vi "Straighten Array.vi"(8 "Error In":errorcluster, 11 "Array":dbl[](array[numeric])) -> (0 "Error Out":errorcluster, 3 "Straightened Array":dbl[](array[numeric]))   [LabVIEW 2021, in "Arrays.lvlib"]
doc: "Tries to make consecutive values monotonically increasing.\nWill fail if the last value is not the larges one."
uses:
  Arrays.lvlib
panel:
  out "Waveform Chart":T1(graph)
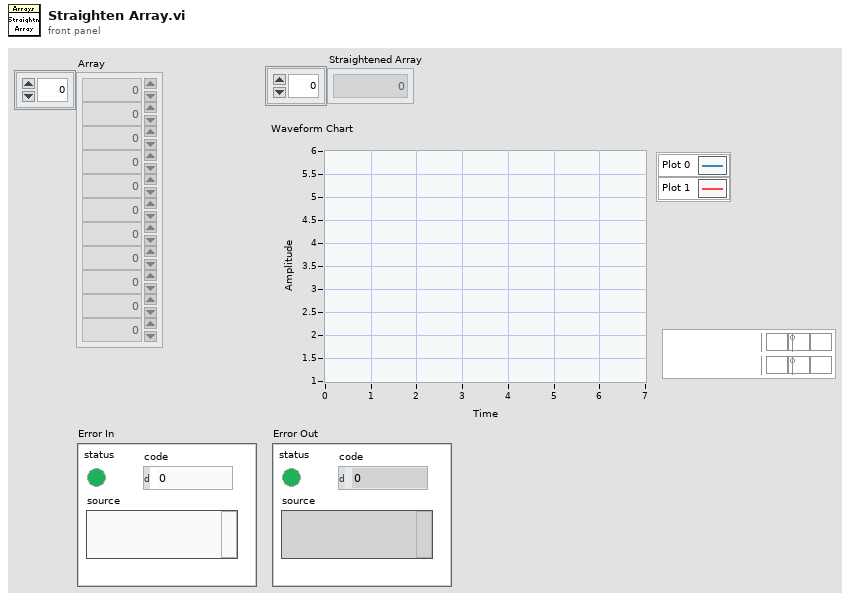
[diagram p1: front panel]
types:
  T1 = cluster{"Numeric Control":dbl, "Numeric Control":dbl}
  T2 = cluster{"Numeric Control":dbl, "Numeric Control":dbl}[]
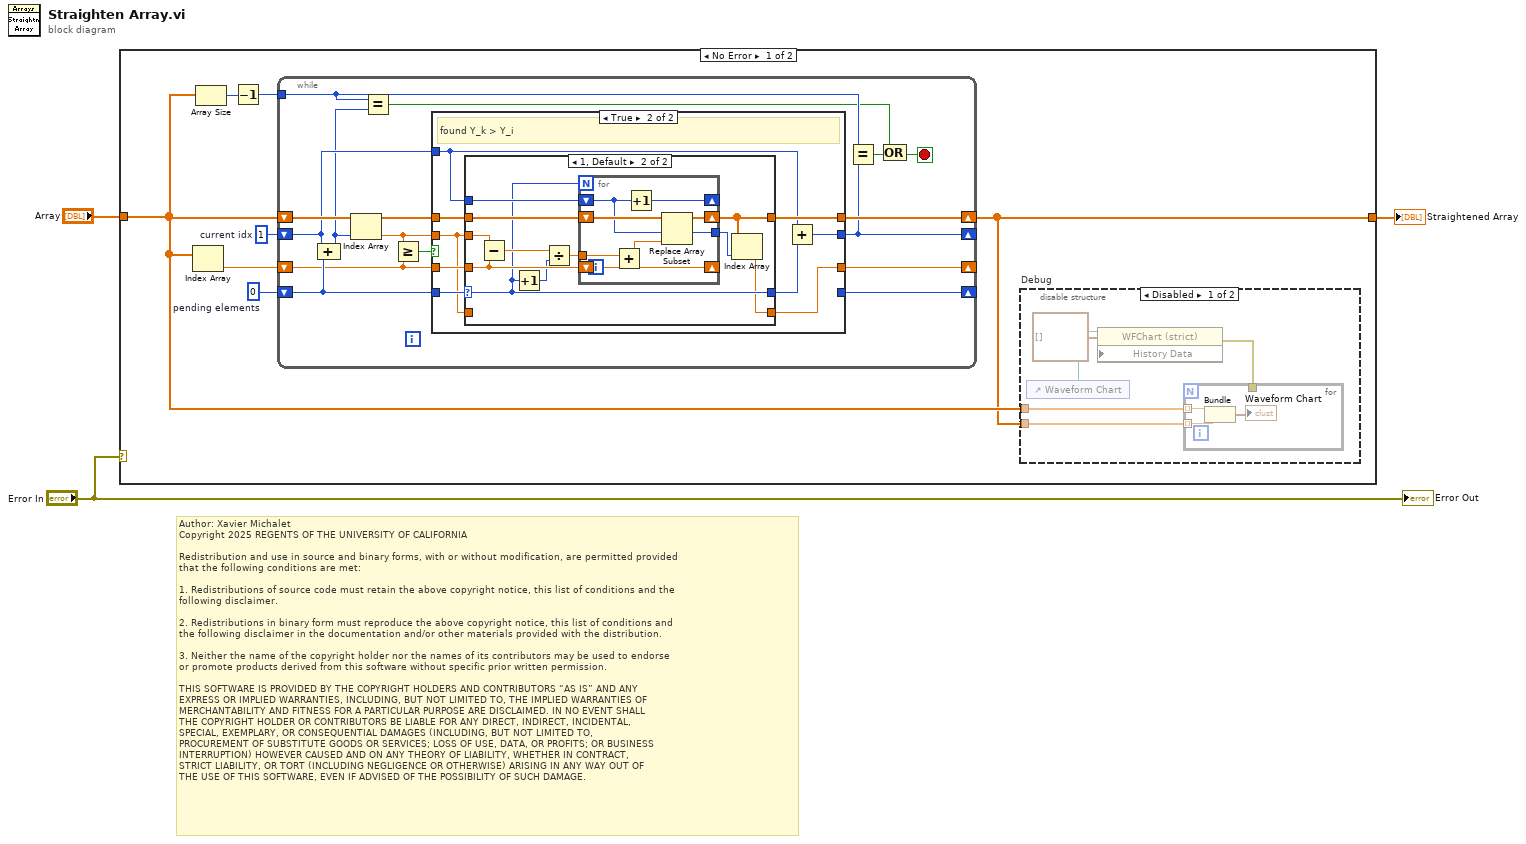
[diagram p0: block diagram]
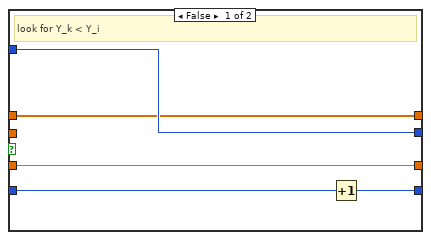
[diagram p2: hidden frame]
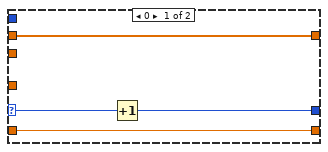
[diagram p3: hidden frame]
diagram:
  # "Author: Xavier Michalet\nCopyright 2025 REGENTS OF THE UNIVERSITY OF CALIFORNIA\n\nRedistribution and use in source and binary forms, with or without modification, are permitted provided\nthat the following conditions are met:\n\n1. Redistributions of source code must retain the above copyright notice, this list of conditions and the\nfollowing disclaimer.\n\n2. Redistributions in binary form must reproduce the above copyright notice, this list of conditions and\nthe following disclaimer in the documentation and/or other materials provided with the distribution.\n\n3. Neither the name of the copyright holder nor the names of its contributors may be used to endorse \nor promote products derived from this software without specific prior written permission.\n\nTHIS SOFTWARE IS PROVIDED BY THE COPYRIGHT HOLDERS AND CONTRIBUTORS “AS IS” AND ANY \nEXPRESS OR IMPLIED WARRANTIES, INCLUDING, BUT NOT LIMITED TO, THE IMPLIED WARRANTIES OF\nMERCHANTABILITY AND FITNESS FOR A PARTICULAR PURPOSE ARE DISCLAIMED. IN NO EVENT SHALL\nTHE COPYRIGHT HOLDER OR CONTRIBUTORS BE LIABLE FOR ANY DIRECT, INDIRECT, INCIDENTAL, \nSPECIAL, EXEMPLARY, OR CONSEQUENTIAL DAMAGES (INCLUDING, BUT NOT LIMITED TO, \nPROCUREMENT OF SUBSTITUTE GOODS OR SERVICES; LOSS OF USE, DATA, OR PROFITS; OR BUSINESS\nINTERRUPTION) HOWEVER CAUSED AND ON ANY THEORY OF LIABILITY, WHETHER IN CONTRACT, \nSTRICT LIABILITY, OR TORT (INCLUDING NEGLIGENCE OR OTHERWISE) ARISING IN ANY WAY OUT OF\nTHE USE OF THIS SOFTWARE, EVEN IF ADVISED OF THE POSSIBILITY OF SUCH DAMAGE."
  n1 = case shown="No Error" "Error In" {
    tunnel: "Array" -> [w7 w70]
    tunnel: [w6 w70] -> w2
    frame No Error {
      w8 = 0  # pending elements
      w9 = 1  # current idx
      n2 = Index Array(array=w7) -> (element=w10:dbl)  [unwired: 1 in]
      n3 = Array Size(array=w7) -> (size(s)=w5:i32)
      n4 = Decrement(x=w5) -> (x-1=w4:i32)
      n5 = while {
        shift-right: [w18] -> w6
        shift-left: w7 -> [w19]
        shift-right: [w17] -> _
        shift-left: w9 -> [w16]
        shift-right: [w24] -> _
        shift-left: w10 -> [w20]
        shift-right: [w22] -> _
        shift-left: w8 -> [w21]
        tunnel: w4 -> [w14]
        stop <- w13 stop-if-true
        n6 = Compound Arithmetic op=ADD(w16, w21) -> (w15:i32)
        n7 = Index Array(array=w19, index=w15) -> (element=w23:dbl)
        n8 = Equal?(x=w14, y=w15) -> (x = y?=w11:bool)
        n9 = Greater Or Equal?(x=w23, y=w20) -> (x >= y?=w25:bool)
        n10 = case shown="True" w25 {
          tunnel: w16 -> [w29 w35]
          tunnel: [w29 w33] -> w17
          tunnel: [w28 w31] -> w24
          tunnel: w23 -> [_ w32]
          tunnel: [w27 _] -> w22
          tunnel: w21 -> [w30 w39]
          tunnel: w20 -> [w28 w36]
          tunnel: w19 -> [w26 w38]
          tunnel: [w26 w37] -> w18
          frame False {
            # "look for Y_k < Y_i"
            n11 = Increment(x=w30) -> (x+1=w27:i32)
          }
          frame True {
            # "found Y_k > Y_i"
            n12 = case shown="1, Default" w39 {
              selector: w39 -> [w42 w47]
              tunnel: w38 -> [w43 w54]
              tunnel: [w43 w46] -> w37
              tunnel: w32 -> [_ w53]
              tunnel: w36 -> [_ w52]
              tunnel: w35 -> [_ w51]
              tunnel: [w41 w47] -> w34
              tunnel: w32 -> [w40 _]
              tunnel: [w40 w44] -> w31
              frame 0 {
                n13 = Increment(x=w42) -> (x+1=w41:i32)
              }
              frame 1, Default {
                n14 = Subtract(x=w53, y=w52) -> (x-y=w50:dbl)
                n15 = Increment(x=w47) -> (x+1=w48:i32)
                n16 = Divide(x=w50, y=w48) -> (x/y=w49:dbl)
                n17 = for {
                  N: w47 -> [_]
                  shift-right: [w59] -> w46
                  shift-left: w54 -> [w60]
                  shift-right: [w58] -> _
                  shift-left: w51 -> [w55]
                  shift-right: [w57] -> _
                  shift-left: w52 -> [w61]
                  tunnel: w49 -> [w56]
                  tunnel: [w55] -> w45
                  n18 = Add(x=w56, y=w61) -> (x+y=w57:dbl)
                  n19 = Increment(x=w55) -> (x+1=w58:i32)
                  n20 = Replace Array Subset(array=w60, new element=w57, index=w55) -> (w59:dbl[])
                }
                n21 = Index Array(array=w46, index=w45) -> (element=w44:dbl)
              }
            }
            n22 = Add(x=w35, y=w34) -> (x+y=w33:i32)
          }
        }
        n23 = Equal?(x=w14, y=w17) -> (x = y?=w12:bool)
        n24 = Compound Arithmetic op=OR(w11, w12) -> (w13:bool)
      }
      n25 = disable-structure "Debug" shown="Disabled" {
        disable-tunnel: w7 -> [w66 _]
        disable-tunnel: w6 -> [w65 _]
        frame Disabled {
          n26 = control-ref of="Waveform Chart"() -> (w64:refnum<vi>)
          n27 = property class="WFChart (strict)"(reference=w64, "History Data"=T2 []) -> (error out=w62:errorcluster)  [unwired: 1 in, 1 out]
          n28 = for {
            tunnel: w66 -> [w69] mode=indexing
            tunnel: w65 -> [w68] mode=indexing
            tunnel: w62 -> [_]
            n29 = Bundle("Numeric Control"=w69, "Numeric Control"=w68) -> (→"Waveform Chart":T1)  [unwired: 1 in]
          }
        }
        frame Enabled {
        }
      }
    }
    frame Error {
    }
  }
  "Straightened Array" <- w2
  "Error Out" <- "Error In"
